vi "Calibration_user_input.vi"(4 "data mode":enum16{"Take new data point", "Refit Curve"}(ring), 6 "Mode":T5, 7 "Fixed n":bool, 8 "OK":T12, 9 "Sampling speeds":T6={"Samples /ch"=300, "Sampling Rate /ch (Hz)"=50.0} {"Sampling Rate /ch (Hz)" min=0 format="%.2f"; "Samples /ch" min=0 step=1}) -> (0 "Ch & Spans":T1[](array[typedef]) {"Ch No" min=0 max=7; "low limit (-10V)" min=-10 max=10 format="%.3f"; "high limit (10V)" min=-10 max=10 format="%.3f"}, 1 "Sampling speeds Output":T6={"Samples /ch"=300, "Sampling Rate /ch (Hz)"=50.0} {"Sampling Rate /ch (Hz)" min=0 format="%.2f"; "Samples /ch" min=0 step=1}, 2 "Fixed n out":bool, 3 "Temp (deg C)":dbl=21.0 format="%.1f", 5 "Abs Press (mbar)":dbl=1013.0 format="%.1f")   [LabVIEW 2013]
uses:
  Controls/ok_button.ctl
  Controls/TypeCalib.ctl
  Controls/Cal_Inst_type.ctl
  Controls/Calibration.ctl
  Calib_setup.ctl
  Controls/Ref_Inst_type.ctl
  Calib_mode.ctl
  Controls/PWA_Data.ctl
  File/Setup_Filetype.ctl
  Controls/Inst_type.ctl
  ADAM Client/Sub VIs/ADAM Controls/Channel_names.ctl
  Controls/LDA_Setup.ctl
  Controls/Setup.ctl
  Globals/Calib_global.vi
  Globals/Meas_global.vi
  Globals/LDA_meas_global_1.vi
  Globals/LDA_meas_global_2.vi
panel:
  in  "Acquisition Plug in":u16(ring) items=["ADAM_Server_Channels.vi", "Channels_and_Index.ctl", "DataTranslation.vi", "DT_With_Multiplexer.vi", "LDA_IP.vi", "NI-DAQmx.vi", "Simulate_kernal.vi"]
  in  "PWA Data":T2
  in  "Preston tube diammeter in mm":dbl min=0.0
  in  "Reference instrument Orig":T4={"high limit (10V)"=4.0, "low limit (-10V)"=0.0, "Ch No"=4, "Off ch no"=0, "Calib filename"=path "", "Ref Instrument type"=enum."Enter Value"} {"Off ch no" min=0 max=1; "Ch No" min=0 max=7; "low limit (-10V)" min=-10 max=10 format="%.1f"; "high limit (10V)" min=-10 max=10 format="%.1f"}
  out "Message":string
  in  "Ref Instrument type":T3
  out "Info":string
  out "XW Angle Calib Present?":bool
  out "XW Velocity Calib Present?":bool
  in  "Edit temp and Press":bool
  out "2nd ref instrument":T7={"2nd Ref type"=enum."LDA", "2nd inst present"=TRUE}
  in  "Ref vel for angle calib":T8={"high limit (10V)"=6.0, "low limit (-10V)"=0.0, "Ch No"=4, "Off ch no"=0, "Calib filename"=path "", "Ref Instrument type"=enum."LDA", "DAQmx Channel"=""} {"Off ch no" min=0 max=1; "Ch No" min=0 max=50; "low limit (-10V)" min=-10 max=10 format="%.1f"; "high limit (10V)" min=-10 max=10 format="%.1f"}
  out "Instrument type":T9=enum."Cross wire angle"
  in  "angle calib":T10(ring)
  in  "Reference instrument":T8={"high limit (10V)"=4.0, "low limit (-10V)"=0.0, "Ch No"=4, "Off ch no"=0, "Calib filename"=path "", "Ref Instrument type"=enum."Enter Value", "DAQmx Channel"=""} {"Off ch no" min=0 max=1; "Ch No" min=0 max=50; "low limit (-10V)" min=-10 max=10 format="%.1f"; "high limit (10V)" min=-10 max=10 format="%.1f"}
  in  "instrument to calibrate":T11=[{"high limit (10V)"=5.0, "low limit (-10V)"=3.0, "Ch No"=1, "Off ch no"=1, "DAQmx Channel"=""}, {"high limit (10V)"=5.0, "low limit (-10V)"=3.0, "Ch No"=2, "Off ch no"=1, "DAQmx Channel"=""}] {"Off ch no" min=0 max=1; "Ch No" min=0 max=1000; "low limit (-10V)" min=-10 max=10 format="%.3f"; "high limit (10V)" min=-10 max=10 format="%.3f"}
  in  "Instrument type":T9=enum."Pressure Transducer"
  out "Calib filename":path
  in  "Type":T1={"high limit (10V)"=4.0, "low limit (-10V)"=0.0, "Ch No"=4, "Var name"="LDA", "DAQmx Chan"=""} {"Ch No" min=0 max=7; "low limit (-10V)" min=-10 max=10 format="%.3f"; "high limit (10V)" min=-10 max=10 format="%.3f"}
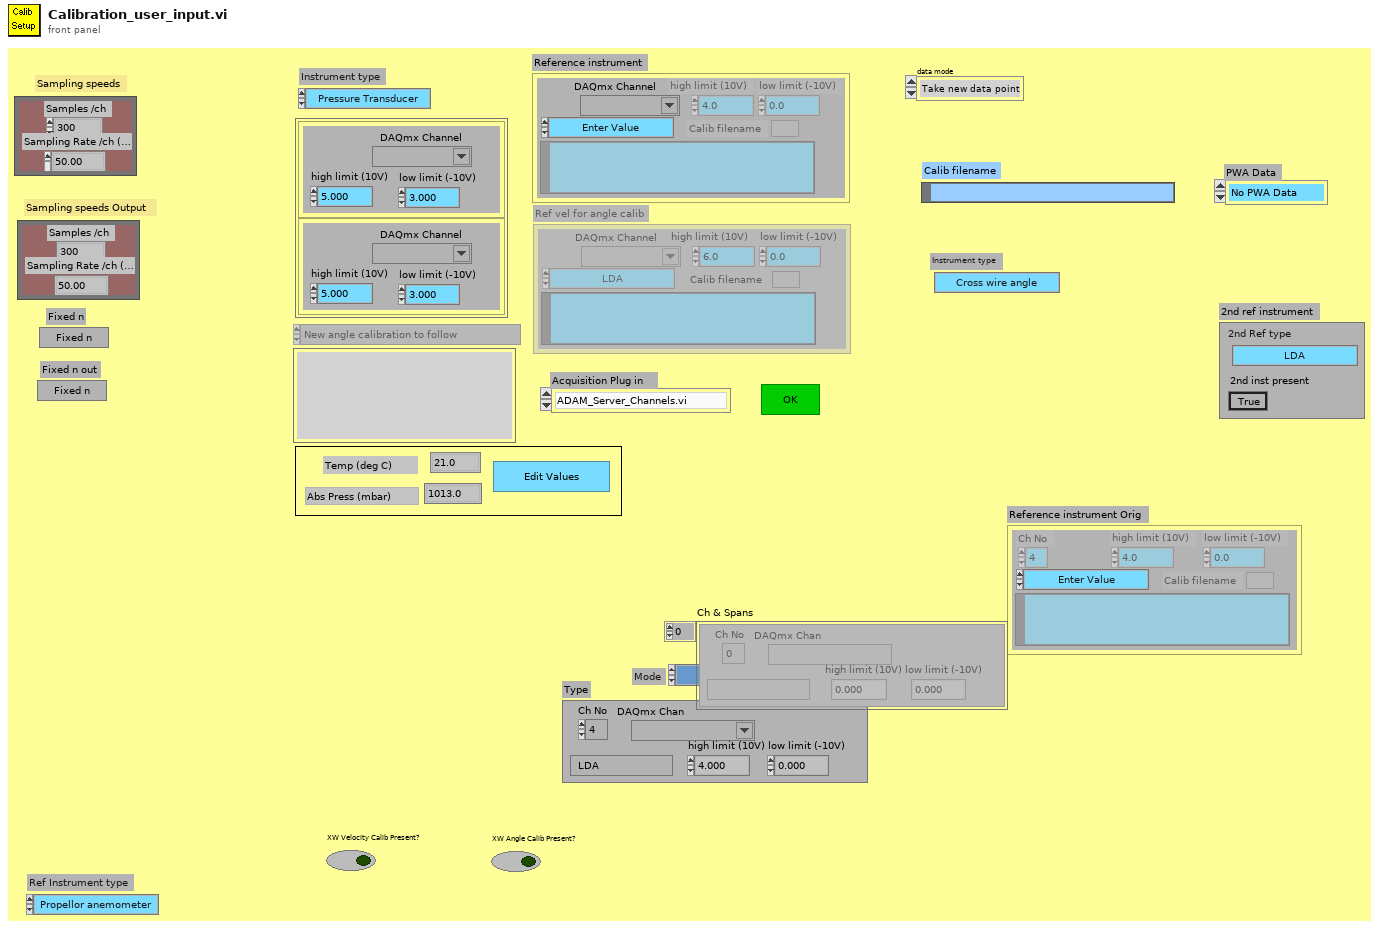
[diagram p1: front panel]
types:
  T1 = typedef "TypeCalib.ctl" = cluster{"high limit (10V)":sgl, "low limit (-10V)":sgl, "Ch No":i16, "Var name":string, "DAQmx Chan":tag}
  T2 = typedef "PWA_Data.ctl" = enum16{"No PWA Data", "One Ch PWA"}
  T3 = typedef "Ref_Inst_type.ctl" = enum16{"Propellor anemometer", "Pressure Transducer", "Raw voltage", "Pitot-static tube", "Preston tube", "Generic Linear", "Generic Polynomial", "Thermocouple", "LDA", "Enter Value", "ADAM Channel"}
  T4 = cluster{"high limit (10V)":sgl, "low limit (-10V)":sgl, "Ch No":i16, "Off ch no":i8, "Calib filename":path, "Ref Instrument type":T3}
  T5 = typedef "Calib_mode.ctl" = enum16{"Show Setup", "Take a New Calibration Point", "Refit Curve", "Setup Front Panel"}
  T6 = cluster{"Samples /ch":i32, "Sampling Rate /ch (Hz)":sgl}
  T7 = cluster{"2nd Ref type":T3, "2nd inst present":bool}
  T8 = typedef "Calib_setup.ctl" = cluster{"high limit (10V)":sgl, "low limit (-10V)":sgl, "Ch No":i16, "Off ch no":i8, "Calib filename":path, "Ref Instrument type":T3, "DAQmx Channel":tag}
  T9 = typedef "Cal_Inst_type.ctl" = enum16{"Propeller anemometer", "Pressure Transducer", "Hot wire", "Cross wire velocity", "Cross wire angle", "Generic Linear", "Generic Polynomial", "Generic BackPoly", "Fast FID", "Thermocouple", "Cold wire", "Pulsed Wire"}
  T10 = enum16{"New angle calibration to follow", "Use the most recent angle calibration"}
  T11 = typedef "Calibration.ctl" = cluster{"high limit (10V)":sgl, "low limit (-10V)":sgl, "Ch No":i16, "Off ch no":i8, "DAQmx Channel":tag}[]
  T12 = typedef "ok_button.ctl" = bool
  T13 = typedef "Setup_Filetype.ctl" = enum16{"Measurement Setups", "Calibration Setups", "General", "Results File Plotter Setups", "Speed Calib Tweaks"}
  T14 = typedef "Inst_type.ctl" = enum16{"Propeller anemometer", "Raw voltage", "Pressure Transducer", "Pitot-static tube", "Preston tube", "Hot wire", "Cross wire 1", "Cross wire 2", "Generic Linear", "Generic Polynomial", "Generic BackPoly", "Fast FID", "Thermocouple", "Cold wire", "Pulsed Wire", "LDA Vel", "LDA Tran time", "LDA Arr time"}
  T15 = typedef "Channel_names.ctl" = enum16{"Active Only", "Active + Off", "All Channels"}
  T16 = typedef "LDA_Setup.ctl" = cluster{"dimensions":enum16{"1D", "2D"}, "Analogue Freq Multiplier":dbl}
  T17 = typedef "Setup.ctl" = enum16{"Run Program", "Show Setup", "Save Current Setup", "Setup Front Panel"}
  T18 = cluster{"high limit (10V)":sgl, "low limit (-10V)":sgl, "Ch No":i16, "Off ch no":i8, "DAQmx Channel":tag}
  T19 = typedef "BSA_Type.ctl" = enum16{"57N11", "BSA F60"}
  T20 = typedef "BSA_info_Cluster.ctl" = cluster{"GPIB Address":string, "No of Check Bytes":i32, "Extra Info":string, "COLOUR":u32, "Wavelength (nm)":dbl}
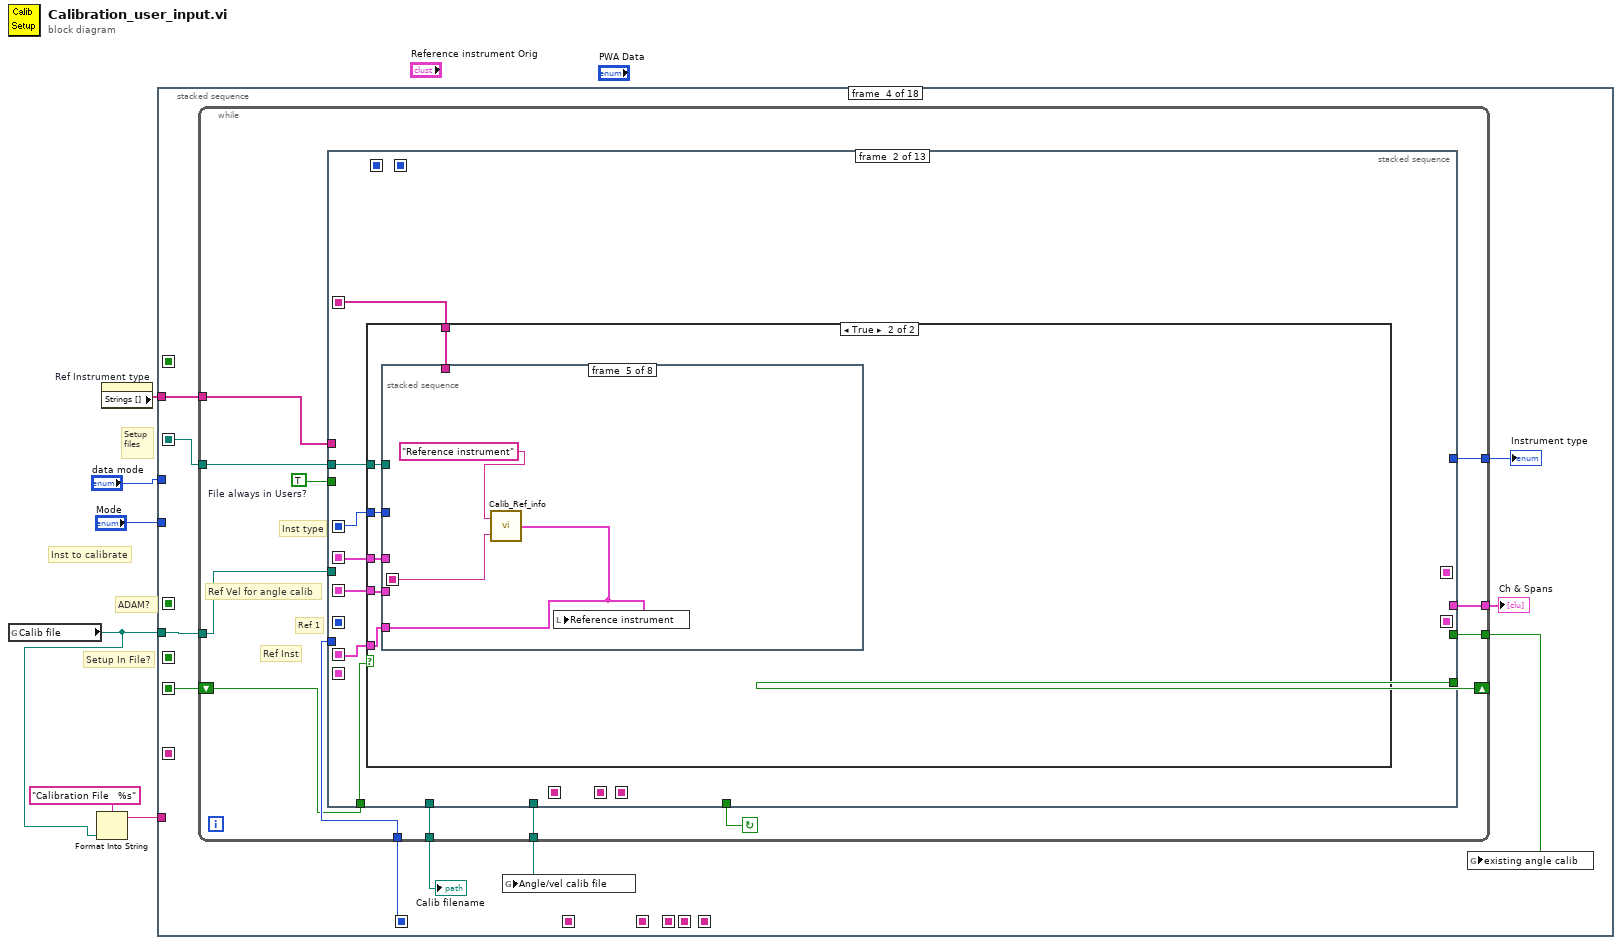
[diagram p0: block diagram]
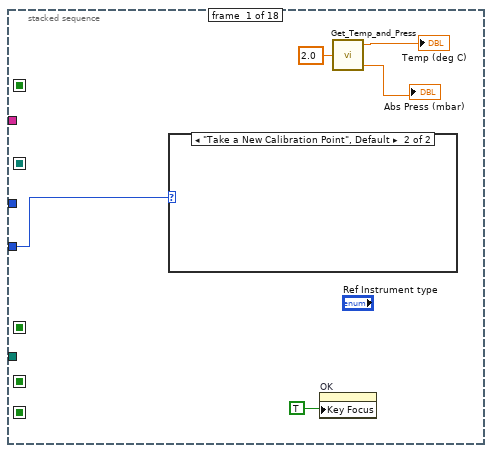
[diagram p2: hidden frame]
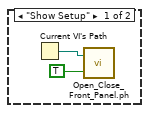
[diagram p3: hidden frame]
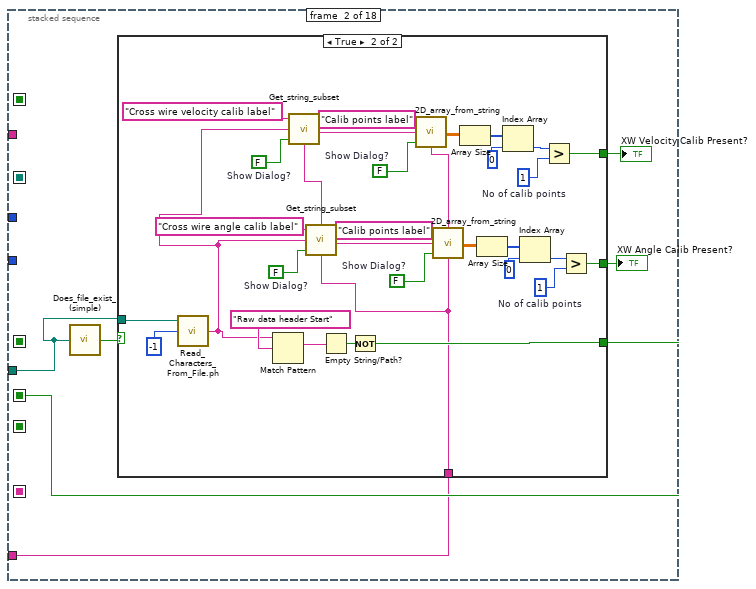
[diagram p4: hidden frame]
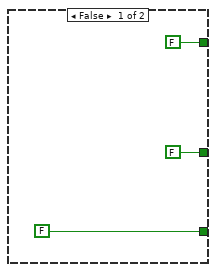
[diagram p5: hidden frame]
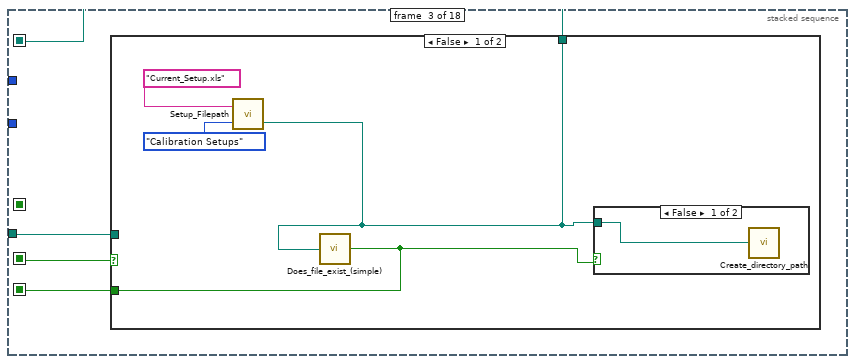
[diagram p6: hidden frame]
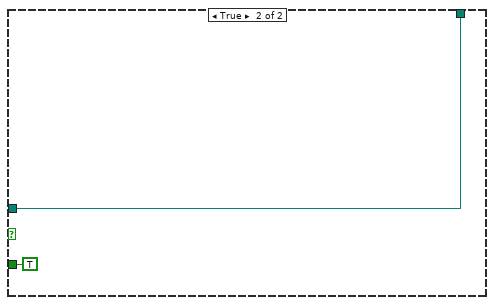
[diagram p8: hidden frame]
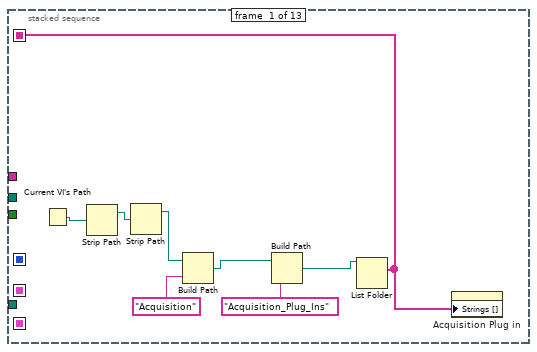
[diagram p9: hidden frame]
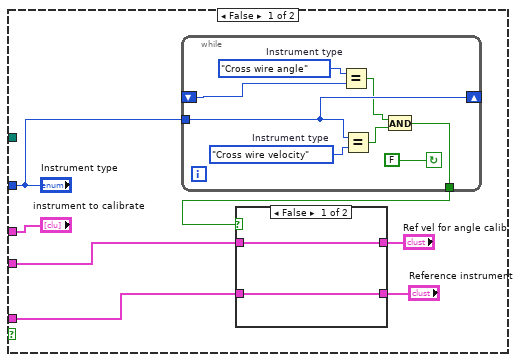
[diagram p10: hidden frame]
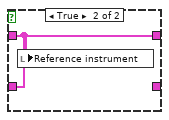
[diagram p11: hidden frame]
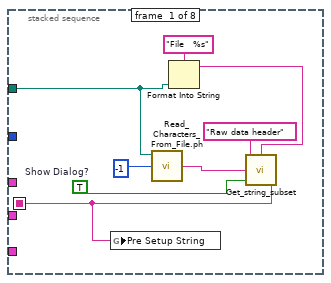
[diagram p12: hidden frame]
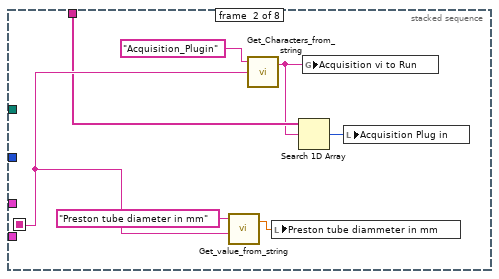
[diagram p13: hidden frame]
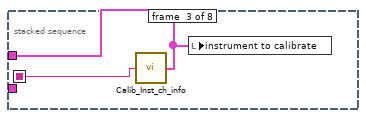
[diagram p14: hidden frame]
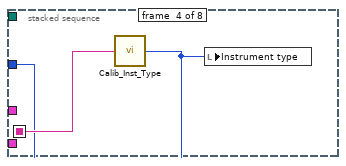
[diagram p15: hidden frame]
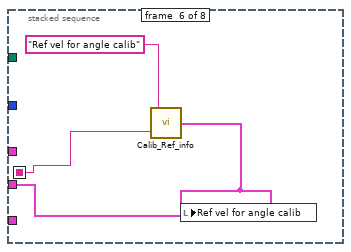
[diagram p16: hidden frame]
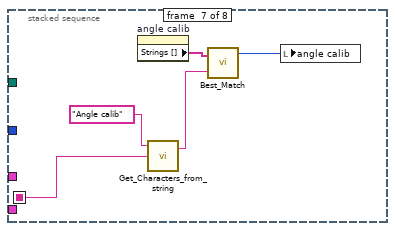
[diagram p17: hidden frame]
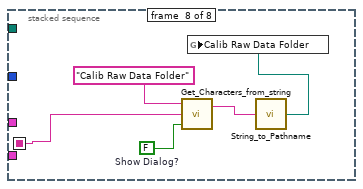
[diagram p18: hidden frame]
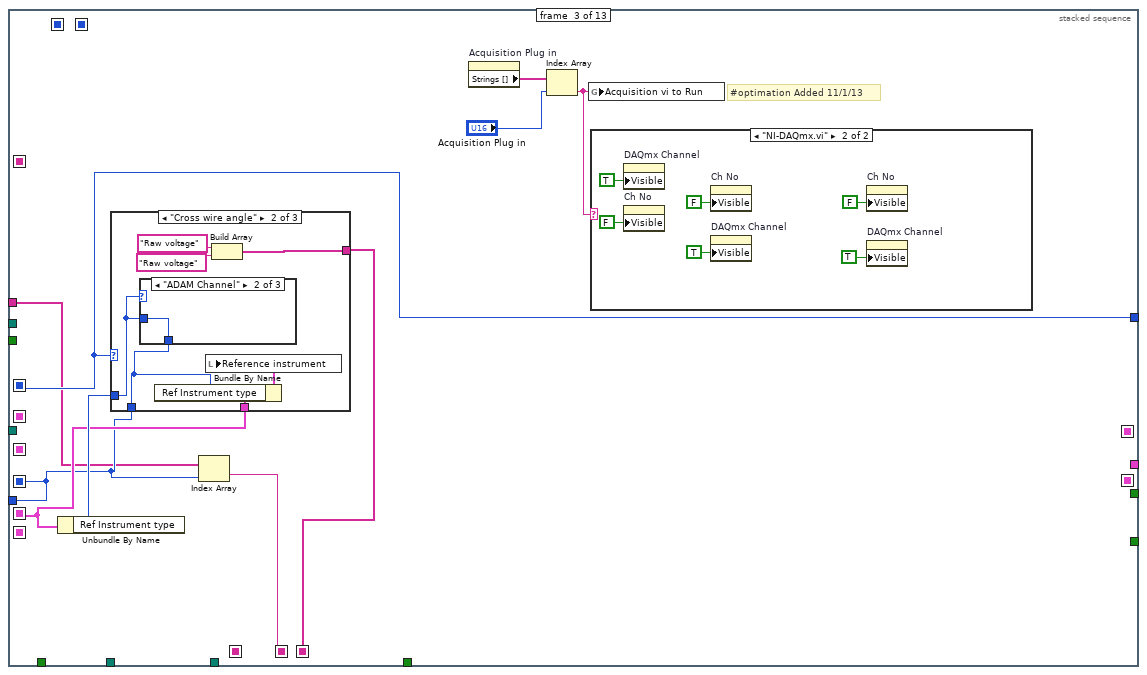
[diagram p19: hidden frame]
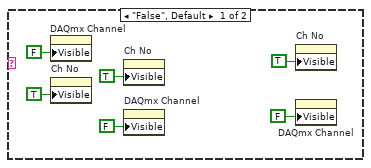
[diagram p20: hidden frame]
diagram:
  # "Inst to calibrate"
  # "Setup In File?"
  # "Setup\nfiles"
  # "ADAM?"
  n1 = global read "Calib_global.vi" "Calib file"() -> (w2:path)
  n2 = Format Into String(format string="Calibration File   %s", w2) -> (resulting string=w1:string)  [unwired: 2 in, 1 out]
  n3 = property on="Ref Instrument type" class="Enum (strict)"() -> ("Strings []"=w4:string[])  [unwired: 2 in, 2 out]
  n4 = stacked-sequence {
    seq-local: [_ _ w55 _ _ _ _ _ _ _ _ _ _ _ _ _ _ _] -> [_ _ _ w72 _ _ _ _ _ _ _ _ _ _ _ _ _ _]
    seq-local: [_ _ w56 _ _ _ _ _ _ _ _ _ _ _ _ _ _ _] -> [_ _ _ w70 _ _ _ _ _ _ _ _ _ _ _ _ _ _]
    seq-local: [_ _ _ w69 _ _ _ _ _ _ _ _ _ _ _ _ _ _] -> [_ _ _ _ _ _ _ w627 _ _ _ _ _ _ _ _ _ _]
    seq-local: [_ _ _ _ _ _ _ w628 _ _ _ _ _ _ _ _ _ _] -> [_ _ _ _ _ _ _ _ w645 _ _ _ _ _ _ _ _ _]
    seq-local: [_ _ _ _ _ _ _ _ w648 _ _ _ _ _ _ _ _ _] -> [_ _ _ _ _ _ _ _ _ _ _ _ _ _ w828 _ _ _]
    seq-local: [_ _ _ _ _ _ _ _ _ _ w737 _ _ _ _ _ _ _] -> [_ _ _ _ _ _ _ _ _ _ _ _ _ _ w827 _ w865 _]
    seq-local: [_ _ _ _ _ _ _ _ _ _ w734 _ _ _ _ _ _ _] -> [_ _ _ _ _ _ _ _ _ _ _ _ _ _ _ w834 _ _]
    seq-local: [_ w19 _ _ _ _ _ _ _ _ _ _ _ _ _ _ _ _] -> [_ _ w54 _ _ _ _ _ _ _ _ _ _ _ _ _ _ _]
    seq-local: [_ _ _ _ _ _ _ _ _ _ _ w749 _ _ _ _ _ _] -> [_ _ _ _ _ _ _ _ _ _ _ _ _ _ w820 _ _ _]
    seq-local: [_ _ _ _ _ _ _ _ _ _ _ _ _ w774 _ _ _ _] -> [_ _ _ _ _ _ _ _ _ _ _ _ _ _ w808 _ _ _]
    seq-local: [_ _ _ _ _ _ _ _ _ _ _ _ w756 _ _ _ _ _] -> [_ _ _ _ _ _ _ _ _ _ _ _ _ _ w804 _ w856 _]
    seq-local: [_ _ _ _ _ _ _ _ _ w683 _ _ _ _ _ _ _ _] -> [_ _ _ _ _ _ _ _ _ _ _ _ _ _ w803 _ _ _]
    tunnel: "Mode" -> [w7 _ _ _ w550 w568 _ _ w647 w696 _ _ w757 _ _ w836 _ w882]
    tunnel: "data mode" -> [_ _ _ _ w544 _ _ _ _ _ _ _ _ _ _ _ _ _]
    tunnel: w2 -> [_ w17 w53 w66 _ _ _ _ _ _ _ _ _ _ _ _ _ _]
    tunnel: w4 -> [_ _ _ w65 _ _ _ _ _ _ _ _ _ _ _ _ _ _]
    tunnel: w1 -> [_ w14 _ _ _ _ _ _ _ _ _ _ _ _ _ _ _ _]
    frame #0 {
      n5 = case shown="\"Take a New Calibration Point\", Default" w7 {
        frame "Show Setup" {
          n6 = Current VI's Path() -> (path=w13:path)
          n7 = call "Open_Close_Front_Panel.ph.vi"("Front Panel Window:Open"=TRUE, "VI path"=w13) -> ()  [unwired: 2 out]
        }
        frame "Take a New Calibration Point", Default {
        }
      }
      n8 = property on="OK" class="Bool"("Key Focus"=TRUE) -> ()  [unwired: 2 in, 2 out]
      n9 = call "Get_Temp_and_Press.vi"("Averaging time (mins)"=2.0) -> ("Abs Press (mbar)"=→"Abs Press (mbar)":dbl, "Temperature"=→"Temp (deg C)":dbl)  [unwired: 3 out]
    }
    frame #1 {
      n10 = call "Does_file_exist_(simple).vi"("Pathname"=w17) -> ("exists?"=w18:bool)
      n11 = case shown="True" w18 {
        tunnel: [FALSE w48] -> w19
        tunnel: w17 -> [_ w47]
        tunnel: [FALSE w25] -> w16
        tunnel: [FALSE w24] -> w15
        tunnel: w14 -> [_ w23]
        frame False {
        }
        frame True {
          w36 = 1  # No of calib points
          w30 = FALSE  # Show Dialog?
          w28 = FALSE  # Show Dialog?
          w37 = 1  # No of calib points
          w43 = FALSE  # Show Dialog?
          w45 = FALSE  # Show Dialog?
          n12 = call "Read_Characters_From_File.ph.vi"("file path (dialog if empty)"=w47, "number of characters (all:-1)"=-1) -> ("character string"=w26:string)  [unwired: 7 out]
          n13 = Match Pattern(string=w26, regular expression="Raw data header Start") -> (match substring=w50:string)  [unwired: 4 out]
          n14 = call "Get_string_subset.vi"("String Name"=w23, "Show Dialog?"=w28, "String to split"=w26, "File Label"="Cross wire velocity calib label") -> ("Output string"=w34:string)  [unwired: 1 out]
          n15 = call "Get_string_subset.vi"("String Name"=w23, "Show Dialog?"=w45, "String to split"=w26, "File Label"="Cross wire angle calib label") -> ("Output string"=w39:string)  [unwired: 1 out]
          n16 = Empty String/Path?(string/path=w50) -> (empty?=w49:bool)
          n17 = Not(x=w49) -> (.not. x?=w48:bool)
          n18 = call "2D_array_from_string.vi"("String Name"=w23, "Show Dialog?"=w30, "Input string"=w34, "Array title"="Calib points label") -> ("2D data array"=w31:dbl[][])
          n19 = call "2D_array_from_string.vi"("String Name"=w23, "Show Dialog?"=w43, "Input string"=w39, "Array title"="Calib points label") -> ("2D data array"=w42:dbl[][])
          n20 = Array Size(array=w31) -> (size(s)=w32:i32[])
          n21 = Array Size(array=w42) -> (size(s)=w41:i32[])
          n22 = Index Array(array=w32, index=0 ("Index")) -> (element=w35:i32)
          n23 = Index Array(array=w41, index=0 ("Index")) -> (element=w38:i32)
          n24 = Greater?(x=w35, y=w36) -> (0:w24:bool)
          n25 = Greater?(x=w38, y=w37) -> (0:w25:bool)
        }
      }
      "XW Velocity Calib Present?" <- w15
      "XW Angle Calib Present?" <- w16
    }
    frame #2 {
      n26 = case shown="False" w54 {
        tunnel: [w60 TRUE ("exists")] -> w56
        tunnel: [w57 w63] -> w55
        tunnel: w53 -> [_ w63]
        frame False {
          n27 = call "Setup_Filepath.vi"("Setup File Type"=Setup_Filetype."Calibration Setups", "Filename in"="Current_Setup.xls") -> ("Filename Out"=w57:path)  [unwired: 1 out]
          n28 = call "Does_file_exist_(simple).vi"("Pathname"=w57) -> ("exists?"=w60:bool)
          n29 = case shown="False" w60 {
            tunnel: w57 -> [w61 _]
            frame False {
              n30 = call "Create_directory_path.vi"("Path name"=w61) -> ()  [unwired: 1 in, 2 out]
            }
            frame True {
            }
          }
        }
        frame True {
        }
      }
    }
    frame #3 {
      n31 = while {
        tunnel: w65 -> [w77]
        shift-left: w70 -> [w80]
        shift-right: [w79] -> _
        tunnel: [w81] -> w71
        tunnel: w72 -> [w82]
        tunnel: [w83] -> w68
        tunnel: [w84] -> w64
        tunnel: [w85] -> w69
        tunnel: [w86] -> w73
        tunnel: [w75] -> w67
        tunnel: w66 -> [w74]
        stop <- w78 continue-if-true
        w76 = TRUE  # File always in Users?
        # "Ref 1"
        # "Ref Inst"
        # "Ref Vel for angle calib"
        # "Inst type"
        n32 = stacked-sequence {
          seq-local: [_ _ w166 _ _ _ _ _ _ _ _ _ _] -> [_ _ _ _ _ w294 _ _ _ _ _ _ _]
          seq-local: [_ _ w170 _ _ _ _ _ _ _ _ _ _] -> [_ _ _ _ _ _ _ _ w445 _ _ _ _]
          seq-local: [_ _ _ _ _ w288 _ _ _ _ _ _ _] -> [_ _ _ _ _ _ _ _ _ w463 _ _ _]
          seq-local: [_ _ w165 _ _ _ _ _ _ _ _ _ _] -> [_ _ _ _ _ _ _ _ _ w461 _ _ _]
          seq-local: [_ _ _ _ _ _ _ _ w444 _ _ _ _] -> [_ _ _ _ _ _ _ _ _ w462 _ _ _]
          seq-local: [_ _ _ _ _ _ _ w366 _ _ _ _ _] -> [_ _ _ _ _ _ _ _ _ w458 _ _ _]
          seq-local: [_ _ _ _ _ _ w362 _ _ _ _ _ _] -> [_ _ _ _ _ _ _ _ _ w457 _ _ _]
          seq-local: [_ w99 _ _ _ _ _ _ _ _ _ _ _] -> [_ _ w168 w205 w218 _ _ w367 _ _ _ _ _]
          seq-local: [_ w98 _ _ _ _ _ _ _ _ _ _ _] -> [_ _ _ w204 _ _ _ _ _ _ _ _ _]
          seq-local: [_ w97 _ _ _ _ _ _ _ _ _ _ _] -> [_ _ _ _ _ _ w364 w368 _ w456 _ _ _]
          seq-local: [_ w96 _ _ _ _ _ _ _ _ _ _ _] -> [_ _ w167 _ _ _ _ _ _ w455 _ _ w543]
          seq-local: [_ _ _ _ _ _ _ _ _ w454 _ _ _] -> [_ _ _ _ _ _ _ _ _ _ _ w502 _]
          seq-local: [_ _ _ w200 _ _ _ _ _ _ _ _ _] -> [_ _ _ _ _ _ _ _ w443 _ _ _ _]
          seq-local: [w87 _ _ _ _ _ _ _ _ _ _ _ _] -> [_ w95 _ _ _ _ _ _ _ _ _ _ _]
          tunnel: [_ _ _ _ _ _ _ _ _ w460 _ _ _] -> w86
          tunnel: [_ _ w166 _ _ _ _ _ _ _ _ _ _] -> w85
          tunnel: [_ _ _ _ _ _ _ _ _ w454 _ _ _] -> w84
          tunnel: [_ _ _ _ w223 _ _ _ _ _ _ _ _] -> w83
          tunnel: w82 -> [_ w101 _ _ _ _ _ _ _ _ _ _ _]
          tunnel: [_ _ w168 _ _ _ _ _ _ _ _ _ _] -> w81
          tunnel: w80 -> [_ w100 _ _ _ _ _ _ _ _ _ _ _]
          tunnel: [_ _ _ _ _ _ _ _ _ _ _ FALSE _] -> w79
          tunnel: [_ _ _ _ _ _ _ _ _ _ _ w500 _] -> w78
          tunnel: w77 -> [_ _ w164 _ _ _ w361 _ _ _ _ _ _]
          tunnel: w76 -> [_ _ _ _ _ _ _ _ _ _ _ _ _]
          tunnel: [_ _ _ _ w222 _ _ _ _ _ _ _ _] -> w75
          tunnel: w74 -> [_ _ _ _ w224 _ _ _ _ _ _ _ _]
          frame #0 {
            n33 = Current VI's Path() -> (path=w90:path)
            n34 = Strip Path(path=w90) -> (stripped path=w89:path)  [unwired: 1 out]
            n35 = Strip Path(path=w89) -> (stripped path=w88:path)  [unwired: 1 out]
            n36 = Build Path(base path=w88, name or relative path="Acquisition") -> (appended path=w93:path)
            n37 = Build Path(base path=w93, name or relative path="Acquisition_Plug_Ins") -> (appended path=w94:path)
            n38 = List Folder(path=w94) -> (filenames=w87:string[])  [unwired: 3 in, 3 out]
            n39 = property on="Acquisition Plug in" class="Ring (strict)"("Strings []"=w87) -> ()  [unwired: 2 in, 2 out]
          }
          frame #1 {
            n40 = case shown="True" w100 {
              tunnel: w101 -> [_ w125]
              tunnel: ["Instrument type" w123] -> w99
              tunnel: ["instrument to calibrate" w124] -> w98
              tunnel: [w103 w121] -> w97
              tunnel: [w105 w122] -> w96
              tunnel: w95 -> [_ w120]
              frame False {
                n41 = while {
                  shift-right: [w117] -> _
                  shift-left: _ -> [w115]
                  tunnel: "Instrument type" -> [w117]
                  tunnel: [w112] -> w106
                  stop <- FALSE continue-if-true
                  w116 = Cal_Inst_type."Cross wire angle"  # Instrument type
                  w118 = Cal_Inst_type."Cross wire velocity"  # Instrument type
                  n42 = Equal?(x=w116, y=w115) -> (x = y?=w113:bool)
                  n43 = Equal?(x=w117, y=w118) -> (x = y?=w114:bool)
                  n44 = And(x=w113, y=w114) -> (x .and. y?=w112:bool)
                }
                n45 = case shown="False" w106 {
                  tunnel: [w110 w111] -> w105
                  tunnel: "Reference instrument" -> [w110 _]
                  tunnel: [w109 w111] -> w103
                  tunnel: "Ref vel for angle calib" -> [w109 w111]
                  frame False {
                  }
                  frame True {
                    n46 = local write "Reference instrument"(w111) -> ()
                  }
                }
              }
              frame True {
                n47 = stacked-sequence {
                  seq-local: [w130 _ _ _ _ _ _ _] -> [_ w137 w142 w144 w146 w149 w153 w158]
                  tunnel: w125 -> [w127 _ _ _ _ _ _ _]
                  tunnel: [_ _ w141 _ _ _ _ _] -> w124
                  tunnel: [_ _ _ w143 _ _ _ _] -> w123
                  tunnel: [_ _ _ _ w145 _ _ _] -> w122
                  tunnel: [_ _ _ _ _ w148 _ _] -> w121
                  tunnel: w120 -> [_ w136 _ _ _ _ _ _]
                  frame #0 {
                    w129 = TRUE  # Show Dialog?
                    n48 = call "Read_Characters_From_File.ph.vi"("file path (dialog if empty)"=w127, "number of characters (all:-1)"=-1) -> ("character string"=w133:string)  [unwired: 7 out]
                    n49 = Format Into String(format string="File   %s", w127) -> (resulting string=w126:string)  [unwired: 2 in, 1 out]
                    n50 = call "Get_string_subset.vi"("String Name"=w126, "Show Dialog?"=w129, "String to split"=w133, "File Label"="Raw data header") -> ("Output string"=w130:string)  [unwired: 1 out]
                    n51 = global write "Calib_global.vi" "Pre Setup String"(w130) -> ()
                  }
                  frame #1 {
                    n52 = call "Get_value_from_string.vi"("Input string"=w137, "Variable name"="Preston tube diameter in mm") -> ("Value"=w139:dbl)  [unwired: 1 in, 1 out]
                    n53 = call "Get_Characters_from_string.vi"("Input string"=w137, "Variable name"="Acquisition_Plugin") -> ("Value"=w135:string)  [unwired: 1 in, 1 out]
                    n54 = local write "Preston tube diammeter in mm"(w139) -> ()
                    n55 = Search 1D Array(1D array=w136, element=w135) -> (index of element=w134:i32)  [unwired: 1 out]
                    n56 = global write "Meas_global.vi" "Acquisition vi to Run"(w135) -> ()
                    n57 = local write "Acquisition Plug in"(w134) -> ()
                  }
                  frame #2 {
                    n58 = call "Calib_Inst_ch_info.vi"("Input string"=w142) -> ("instrument to calibrate (new)"=w141:T11)
                    n59 = local write "instrument to calibrate"(w141) -> ()
                  }
                  frame #3 {
                    n60 = call "Calib_Inst_Type.vi"("Input string"=w144) -> ("Instrument type"=w143:T9)
                    n61 = local write "Instrument type"(w143) -> ()
                  }
                  frame #4 {
                    n62 = call "Calib_Ref_info.vi"("Input string"=w146, "Reference Name"="Reference instrument") -> ("Reference instrument"=w145:T8)
                    n63 = local write "Reference instrument"(w145) -> ()
                  }
                  frame #5 {
                    n64 = call "Calib_Ref_info.vi"("Input string"=w149, "Reference Name"="Ref vel for angle calib") -> ("Reference instrument"=w148:T8)
                    n65 = local write "Ref vel for angle calib"(w148) -> ()
                  }
                  frame #6 {
                    n66 = property on="angle calib" class="Enum (strict)"() -> ("Strings []"=w155:string[])  [unwired: 2 in, 2 out]
                    n67 = call "Get_Characters_from_string.vi"("Input string"=w153, "Variable name"="Angle calib") -> ("Value"=w152:string)  [unwired: 1 in, 1 out]
                    n68 = call "Best_Match.vi"("Input String"=w152, "String Options"=w155) -> ("index of element"=w151:i32)  [unwired: 1 out]
                    n69 = local write "angle calib"(w151) -> ()
                  }
                  frame #7 {
                    w159 = FALSE  # Show Dialog?
                    n70 = call "Get_Characters_from_string.vi"("Show Dialog?"=w159, "Input string"=w158, "Variable name"="Calib Raw Data Folder") -> ("Value"=w157:string)  [unwired: 1 out]
                    n71 = call "String_to_Pathname.vi"("Input String"=w157) -> ("path"=w156:path)
                    n72 = global write "Calib_global.vi" "Calib Raw Data Folder"(w156) -> ()
                  }
                }
              }
            }
          }
          frame #2 {
            # "#optimation Added 11/1/13"
            n73 = Unbundle By Name(w167) -> ("Ref Instrument type"=w169:T3)
            n74 = case shown="\"Cross wire angle\"" w168 {
              tunnel: [w185 w193 w198] -> w170
              tunnel: w169 -> [w183 w187 w197]
              tunnel: [w183 w190 w197] -> w166
              tunnel: w167 -> [_ w191 _]
              frame "Cross wire velocity" {
                n75 = Build Array("Raw voltage", "Raw voltage") -> (w185:string[])
              }
              frame "Cross wire angle" {
                n76 = case shown="\"ADAM Channel\"" w187 {
                  tunnel: [w194 w195 Ref_Inst_type."Enter Value" ("Ref Instrument type")] -> w190
                  tunnel: w187 -> [w194 w195 _]
                  frame "Enter Value" {
                  }
                  frame "ADAM Channel" {
                  }
                  frame "LDA", Default {
                  }
                }
                n77 = Bundle By Name(cluster=w191, "Ref Instrument type"=w190) -> (w192:T8)
                n78 = local write "Reference instrument"(w192) -> ()
                n79 = Build Array("Raw voltage", "Raw voltage") -> (w193:string[])
              }
              frame "Generic Linear", Default {
                n80 = Build Array("Raw voltage") -> (w198:string[])
              }
            }
            n81 = Index Array(array=w164, index=w166) -> (element=w165:string)
            n82 = property on="Acquisition Plug in" class="Ring (strict)"() -> ("Strings []"=w163:string[])  [unwired: 2 in, 2 out]
            n83 = Index Array(array=w163, index="Acquisition Plug in") -> (element=w161:string)
            n84 = global write "Meas_global.vi" "Acquisition vi to Run"(w161) -> ()
            n85 = case shown="\"NI-DAQmx.vi\"" w161 {
              frame "False", Default {
                n86 = property on="DAQmx Channel" class="DAQmxName"("Visible"=FALSE) -> ()  [unwired: 2 in, 2 out]
                n87 = property on="Ch No" class="DigNum (strict)"("Visible"=TRUE) -> ()  [unwired: 2 in, 2 out]
                n88 = property on="Ch No" class="DigNum (strict)"("Visible"=TRUE) -> ()  [unwired: 2 in, 2 out]
                n89 = property on="DAQmx Channel" class="DAQmxName"("Visible"=FALSE) -> ()  [unwired: 2 in, 2 out]
                n90 = property on="Ch No" class="DigNum (strict)"("Visible"=TRUE) -> ()  [unwired: 2 in, 2 out]
                n91 = property on="DAQmx Channel" class="DAQmxName"("Visible"=FALSE) -> ()  [unwired: 2 in, 2 out]
              }
              frame "NI-DAQmx.vi" {
                n92 = property on="DAQmx Channel" class="DAQmxName"("Visible"=TRUE) -> ()  [unwired: 2 in, 2 out]
                n93 = property on="Ch No" class="DigNum (strict)"("Visible"=FALSE) -> ()  [unwired: 2 in, 2 out]
                n94 = property on="Ch No" class="DigNum (strict)"("Visible"=FALSE) -> ()  [unwired: 2 in, 2 out]
                n95 = property on="DAQmx Channel" class="DAQmxName"("Visible"=TRUE) -> ()  [unwired: 2 in, 2 out]
                n96 = property on="Ch No" class="DigNum (strict)"("Visible"=FALSE) -> ()  [unwired: 2 in, 2 out]
                n97 = property on="DAQmx Channel" class="DAQmxName"("Visible"=TRUE) -> ()  [unwired: 2 in, 2 out]
              }
            }
          }
          frame #3 {
            n98 = Array Size(array=w204) -> (size(s)=w203:i32)
            n99 = case shown="\"Cross wire angle\"" w205 {
              tunnel: [2 2 1 0] -> w202
              frame "Cross wire velocity" {
              }
              frame "Cross wire angle" {
              }
              frame "Generic Linear", Default {
              }
              frame "Pulsed Wire" {
              }
            }
            n100 = Equal?(x=w202, y=w203) -> (x = y?=w201:bool)
            n101 = case shown="False" w201 {
              tunnel: w202 -> [w211 _]
              tunnel: w204 -> [w207 w213]
              tunnel: [w206 w213] -> w200
              frame False {
                n102 = Index Array(array=w207, index=0) -> (element=w208:T18)
                n103 = Build Array (concatenate)(w207, w208) -> (w210:T11)
                n104 = for {
                  N: w211 -> [_]
                  tunnel: w210 -> [w212] mode=indexing
                  tunnel: [w212] -> w206 mode=indexing
                }
                n105 = local write "instrument to calibrate"(w206) -> ()
              }
              frame True {
              }
            }
          }
          frame #4 {
            n106 = case shown="\"Cross wire angle\"" w218 {
              tunnel: w224 -> [_ w235 w257]
              tunnel: [path "" w236 w258] -> w223
              tunnel: [FALSE w234 w256] -> w222
              tunnel: [w225 w230 w252] -> w221
              tunnel: [w227 w233 w255] -> w220
              tunnel: ["" w232 w253] -> w219
              tunnel: w218 -> [_ w231 w254]
              frame "Propeller anemometer", Default {
                w225 = u8 2  # Disabled
                w227 = u8 2  # Disabled
              }
              frame "Cross wire angle" {
                w230 = u8 0  # Disabled
                w233 = u8 2  # Disabled
                n107 = local read "XW Velocity Calib Present?"() -> (w237:bool)
                n108 = case shown="False" w237 {
                  tunnel: [w241 w251] -> w236
                  tunnel: w235 -> [_ w251]
                  tunnel: [TRUE TRUE] -> w234
                  tunnel: [w239 w249] -> w232
                  tunnel: w231 -> [w238 _]
                  frame False {
                    w245 = 0  # index
                    n109 = local read "instrument to calibrate"() -> (w246:T11)
                    n110 = Index Array(array=w246, index=w245) -> (element=w244:T18)
                    n111 = Unbundle By Name(w244) -> ("Ch No"=w242:i16)
                    n112 = call "XW_file_info.vi"("Instrument type"=w238, "Ch No"=w242) -> ("Filename"=w241:path, "resulting string"=w239:string, "File Exists?"=w240:bool)
                    n113 = case shown="False" w240 {
                      frame False {
                        w247 = Cal_Inst_type."Cross wire velocity"  # Instrument type
                        w248 = "You need to do a velocity calibration before you can do the angle calibration"  # message
                        n114 = local write "Instrument type"(w247) -> ()
                        n115 = One Button Dialog(message=w248) -> ()  [unwired: 2 out]
                      }
                      frame True {
                      }
                    }
                  }
                  frame True {
                    w249 = "Will use the velocity Calibration info already in the Calibration file. "  # resulting string
                  }
                }
              }
              frame "Cross wire velocity" {
                w252 = u8 2  # Disabled
                n116 = local read "XW Angle Calib Present?"() -> (w259:bool)
                n117 = case shown="False" w259 {
                  tunnel: [w268 w287] -> w258
                  tunnel: w257 -> [_ w287]
                  tunnel: [TRUE FALSE] -> _
                  tunnel: [w267 TRUE] -> w256
                  tunnel: [w266 w284] -> w255
                  tunnel: w254 -> [w264 _]
                  tunnel: [w261 w283] -> w253
                  frame False {
                    w272 = 0  # index
                    n118 = local read "instrument to calibrate"() -> (w273:T11)
                    n119 = Index Array(array=w273, index=w272) -> (element=w271:T18)
                    n120 = Unbundle By Name(w271) -> ("Ch No"=w265:i16)
                    n121 = call "XW_file_info.vi"("Instrument type"=w264, "Ch No"=w265) -> ("Filename"=w263:path, "resulting string"=w260:string, "File Exists?"=w262:bool)
                    n122 = case shown="\"New angle calibration to follow\"" "angle calib" {
                      tunnel: [path "" w279] -> w268
                      tunnel: w263 -> [_ w279]
                      tunnel: [FALSE TRUE] -> w267
                      tunnel: ["This XW velocity Calibration MUST be followed by an angle calibration, before XW measurements can be made." w277] -> w261
                      tunnel: w260 -> [_ w277]
                      frame "New angle calibration to follow" {
                      }
                      frame "Use the most recent angle calibration" {
                      }
                    }
                    n123 = case shown="False" w262 {
                      tunnel: [w280 w282] -> w266
                      frame False {
                        w280 = u8 2  # Disabled
                        w281 = T10."New angle calibration to follow"  # angle calib
                        n124 = local write "angle calib"(w281) -> ()
                      }
                      frame True {
                        w282 = u8 0  # Disabled
                      }
                    }
                  }
                  frame True {
                    w283 = "Will use the angle Calibration info already in the Calibration file. "  # resulting string
                    w284 = u8 0  # Disabled
                  }
                }
              }
            }
            "Info" <- w219
            n125 = property on="Ref vel for angle calib" class="Clust (strict)"("Disabled"=w221) -> ()  [unwired: 2 in, 2 out]
            n126 = property on="angle calib" class="Enum (strict)"("Disabled"=w220) -> ()  [unwired: 2 in, 2 out]
          }
          frame #5 {
            n127 = case shown="\"Enter Value\"" w294 {
              tunnel: [u8 0 u8 0 u8 0 u8 0 u8 0 u8 0 u8 0 u8 2 u8 2 u8 2 u8 2] -> w289
              tunnel: [u8 0 u8 0 u8 2 u8 0 u8 0 u8 0 u8 0 u8 2 u8 2 u8 2 u8 2] -> w293
              tunnel: [u8 0 u8 0 u8 0 u8 0 u8 0 u8 0 u8 0 u8 2 u8 2 u8 2 u8 2] -> w292
              tunnel: [u8 0 u8 0 u8 0 u8 0 u8 0 u8 0 u8 0 u8 2 u8 2 u8 2 u8 2] -> w291
              tunnel: [u8 0 u8 0 u8 0 u8 0 u8 0 u8 0 u8 0 u8 2 u8 2 u8 2 u8 2] -> w290
              tunnel: [1 1 1 1 1 1 1 0 0 0 0] -> w288
              frame "Propellor anemometer" {
              }
              frame "Pressure Transducer" {
              }
              frame "Raw voltage" {
              }
              frame "Pitot-static tube" {
              }
              frame "Preston tube" {
              }
              frame "Generic Linear" {
              }
              frame "Generic Polynomial" {
              }
              frame "Thermocouple" {
              }
              frame "LDA" {
              }
              frame "Enter Value" {
              }
              frame "ADAM Channel" {
              }
            }
            n128 = property on="Calib filename" class="Path"("Disabled"=w293) -> ()  [unwired: 2 in, 2 out]
            n129 = property on="Ch No" class="DigNum (strict)"("Disabled"=w292) -> ()  [unwired: 2 in, 2 out]
            n130 = property on="high limit (10V)" class="DigNum (strict)"("Disabled"=w291) -> ()  [unwired: 2 in, 2 out]
            n131 = property on="low limit (-10V)" class="DigNum (strict)"("Disabled"=w290) -> ()  [unwired: 2 in, 2 out]
            n132 = property on="Off ch no" class="DigNum (strict)"("Disabled"=w289) -> ()  [unwired: 2 in, 2 out]
          }
          frame #6 {
            n133 = Unbundle By Name(w364) -> ("Ref Instrument type"=w363:T3)
            n134 = Index Array(array=w361, index=w363) -> (element=w362:string)
          }
          frame #7 {
            n135 = Unbundle By Name(w368) -> ("Ref Instrument type"=w369:T3)
            n136 = case shown="\"Pitot-static tube\"" w369 {
              tunnel: [u8 0 u8 0 u8 0 u8 0 u8 0 u8 0 u8 0 u8 0 u8 2 u8 2 u8 2] -> w370
              tunnel: [u8 0 u8 0 u8 2 u8 0 u8 0 u8 0 u8 0 u8 0 u8 2 u8 2 u8 2] -> w374
              tunnel: [u8 0 u8 0 u8 0 u8 0 u8 0 u8 0 u8 0 u8 0 u8 2 u8 2 u8 2] -> w373
              tunnel: [u8 0 u8 0 u8 0 u8 0 u8 0 u8 0 u8 0 u8 0 u8 2 u8 2 u8 2] -> w372
              tunnel: [u8 0 u8 0 u8 0 u8 0 u8 0 u8 0 u8 0 u8 0 u8 2 u8 2 u8 2] -> w371
              tunnel: [enum16{"No 2nd ref inst", "Add 2nd ref inst"}."Add 2nd ref inst" enum16{"No 2nd ref inst", "Add 2nd ref inst"}."Add 2nd ref inst" enum16{"No 2nd ref inst", "Add 2nd ref inst"}."Add 2nd ref inst" enum16{"No 2nd ref inst", "Add 2nd ref inst"}."Add 2nd ref inst" enum16{"No 2nd ref inst", "Add 2nd ref inst"}."Add 2nd ref inst" enum16{"No 2nd ref inst", "Add 2nd ref inst"}."Add 2nd ref inst" enum16{"No 2nd ref inst", "Add 2nd ref inst"}."Add 2nd ref inst" enum16{"No 2nd ref inst", "Add 2nd ref inst"}."Add 2nd ref inst" enum16{"No 2nd ref inst", "Add 2nd ref inst"}."No 2nd ref inst" enum16{"No 2nd ref inst", "Add 2nd ref inst"}."No 2nd ref inst" enum16{"No 2nd ref inst", "Add 2nd ref inst"}."No 2nd ref inst"] -> w365
              frame "Propellor anemometer" {
              }
              frame "Pressure Transducer" {
              }
              frame "Raw voltage" {
              }
              frame "Pitot-static tube" {
              }
              frame "Preston tube" {
              }
              frame "Generic Linear" {
              }
              frame "Generic Polynomial" {
              }
              frame "Thermocouple" {
              }
              frame "LDA" {
              }
              frame "Enter Value" {
              }
              frame "ADAM Channel" {
              }
            }
            n137 = case shown="\"Cross wire angle\"" w367 {
              tunnel: [w375 enum16{"No 2nd ref inst", "Add 2nd ref inst"}."No 2nd ref inst"] -> w366
              tunnel: w365 -> [w375 _]
              frame "Cross wire angle" {
              }
              frame "Generic Linear", Default {
              }
            }
            n138 = property on="Calib filename" class="Path"("Disabled"=w374) -> ()  [unwired: 2 in, 2 out]
            n139 = property on="low limit (-10V)" class="DigNum (strict)"("Disabled"=w373) -> ()  [unwired: 2 in, 2 out]
            n140 = property on="high limit (10V)" class="DigNum (strict)"("Disabled"=w372) -> ()  [unwired: 2 in, 2 out]
            n141 = property on="Ch No" class="DigNum (strict)"("Disabled"=w371) -> ()  [unwired: 2 in, 2 out]
            n142 = property on="Off ch no" class="DigNum (strict)"("Disabled"=w370) -> ()  [unwired: 2 in, 2 out]
          }
          frame #8 {
            n143 = for {
              tunnel: w445 -> [w453] mode=indexing
              tunnel: [w451] -> w444 mode=indexing
              tunnel: w443 -> [w447] mode=indexing
              n144 = Unbundle By Name(w447) -> ("high limit (10V)"=w450:sgl, "low limit (-10V)"=w449:sgl, "Ch No"=w448:i16, "DAQmx Channel"=w446:tag)
              n145 = Bundle By Name(cluster="Type", "high limit (10V)"=w450, "low limit (-10V)"=w449, "Ch No"=w448, "Var name"=w453, "DAQmx Chan"=w446) -> (w451:T1)
            }
          }
          frame #9 {
            n146 = local read "Type"() -> (w459:T1)
            n147 = case shown="..0" w463 {
              tunnel: [w467 w491] -> w454
              tunnel: w462 -> [w470 w485]
              tunnel: w455 -> [_ w488]
              tunnel: w461 -> [_ w487]
              tunnel: [w469 w490] -> w460
              tunnel: w459 -> [w468 w489]
              tunnel: w456 -> [w464 _]
              tunnel: w458 -> [w466 _]
              tunnel: w457 -> [w465 _]
              frame ..0 {
                n148 = case shown="\"Add 2nd ref inst\"" w466 {
                  tunnel: [w472 w483] -> w467
                  tunnel: w465 -> [_ w482]
                  tunnel: w464 -> [_ w481]
                  tunnel: w468 -> [_ w480]
                  tunnel: [path "" w479] -> w469
                  tunnel: w470 -> [w472 w474]
                  frame "No 2nd ref inst" {
                  }
                  frame "Add 2nd ref inst" {
                    n149 = Unbundle By Name(w481) -> ("high limit (10V)"=w476:sgl, "low limit (-10V)"=w477:sgl, "Ch No"=w478:i16, "Calib filename"=w479:path, "DAQmx Channel"=w473:tag)
                    n150 = Bundle By Name(cluster=w480, "high limit (10V)"=w476, "low limit (-10V)"=w477, "Ch No"=w478, "Var name"=w482, "DAQmx Chan"=w473) -> (w475:T1)
                    n151 = Build Array (concatenate)(w475, w474) -> (w483:T1[])
                  }
                }
              }
              frame 1.. {
                n152 = Unbundle By Name(w488) -> ("high limit (10V)"=w494:sgl, "low limit (-10V)"=w493:sgl, "Ch No"=w492:i16, "Calib filename"=w490:path, "DAQmx Channel"=w484:tag)
                n153 = Bundle By Name(cluster=w489, "high limit (10V)"=w494, "low limit (-10V)"=w493, "Ch No"=w492, "Var name"=w487, "DAQmx Chan"=w484) -> (w486:T1)
                n154 = local write "Type"(w486) -> ()
                n155 = Build Array (concatenate)(w486, w485) -> (w491:T1[])
              }
            }
          }
          frame #10 {
            n156 = case shown="True" "Edit temp and Press" {
              frame False {
              }
              frame True {
                n157 = stacked-sequence {
                  frame #0 {
                    w496 = TRUE  # Wait until done
                    n158 = call "Run_Enter_Temp.vi"("Wait until done"=w496) -> ()  [unwired: 1 out]
                  }
                  frame #1 {
                    n159 = call "Get_Temp_and_Press.vi"("Averaging time (mins)"=0.5) -> ("Abs Press (mbar)"=w498:dbl, "Temperature"=w497:dbl)  [unwired: 3 out]
                    n160 = local write "Abs Press (mbar)"(w498) -> ()
                    n161 = local write "Temp (deg C)"(w497) -> ()
                  }
                }
              }
            }
          }
          frame #11 {
            # "#optimation Should probably also check for duplicate DAQmx Channels"
            n162 = case shown="True" "OK" {
              tunnel: w502 -> [_ w506]
              tunnel: [TRUE w505] -> w500
              frame False {
              }
              frame True {
                n163 = stacked-sequence {
                  seq-local: [w507 _] -> [_ w525]
                  tunnel: w506 -> [w509 w527]
                  tunnel: [_ w523] -> w505
                  frame #0 {
                    n164 = for {
                      shift-right: [w516] -> _
                      shift-left: i16[] [] -> [w515]
                      tunnel: w509 -> [w512] mode=indexing
                      tunnel: [w511] -> w508 mode=indexing
                      n165 = Unbundle By Name(w512) -> ("Ch No"=w513:i16)
                      n166 = Search 1D Array(1D array=w515, element=w513) -> (index of element=w514:i32)  [unwired: 1 out]
                      n167 = Build Array (concatenate)(w515, w513) -> (w516:i16[])
                      n168 = case shown="0, Default" w514 {
                        tunnel: w513 -> [w521 _]
                        tunnel: [w517 FALSE ("true")] -> w511
                        frame 0, Default {
                          n169 = Format Into String(format string="The Ch No %d appears more than once", w521) -> (resulting string=w519:string)  [unwired: 2 in, 1 out]
                          n170 = One Button Dialog(message=w519, button name ("OK")="Ok") -> (true=w517:bool)
                        }
                        frame -1 {
                        }
                      }
                    }
                    n171 = Or Array Elements(Boolean array=w508) -> (logical OR=w507:bool)
                  }
                  frame #1 {
                    n172 = for {
                      tunnel: w527 -> [w533] mode=indexing
                      tunnel: [w532] -> w526 mode=indexing
                      n173 = Unbundle By Name(w533) -> ("high limit (10V)"=w531:sgl, "low limit (-10V)"=w530:sgl, "Ch No"=w528:i16)
                      n174 = Greater Or Equal?(x=w531, y=w530) -> (x >= y?=w529:bool)
                      n175 = case shown="False" w529 {
                        tunnel: [TRUE ("true") FALSE ("true")] -> w532
                        tunnel: w528 -> [w535 _]
                        frame False {
                          n176 = Number To Decimal String(number=w535) -> (decimal integer string=w536:string)  [unwired: 1 out]
                          n177 = Concatenate Strings("Error in input limits for Channel No ", w536) -> (w537:string)
                          n178 = One Button Dialog(message=w537) -> ()  [unwired: 2 out]
                        }
                        frame True {
                        }
                      }
                    }
                    n179 = Or Array Elements(Boolean array=w526) -> (logical OR=w524:bool)
                    n180 = Or(x=w524, y=w525) -> (x .or. y?=w523:bool)
                  }
                }
              }
            }
          }
          frame #12 {
            n181 = Unbundle By Name(w543) -> ("Ref Instrument type"=w542:T3)
            n182 = Equal?(x=Ref_Inst_type."Preston tube" ("Ref Instrument type"), y=w542) -> (x = y?=w540:bool)
            n183 = property on="Preston tube diammeter in mm" class="DigNum (strict)"("Visible"=w540) -> ()  [unwired: 2 in, 2 out]
          }
        }
      }
      "Instrument type" <- w71
      "Calib filename" <- w73
      "Ch & Spans" <- w64
      n184 = global write "Calib_global.vi" "Angle/vel calib file"(w68) -> ()
      n185 = global write "Calib_global.vi" "existing angle calib"(w67) -> ()
    }
    frame #4 {
      n186 = global read "Calib_global.vi" "Pre Setup String"() -> (w545:string)
      n187 = case shown="\"Setup Front Panel\"" w550 {
        tunnel: [w552 w562] -> w549
        tunnel: "Sampling speeds" -> [w552 w564]
        tunnel: [w551 w558] -> w547
        tunnel: "Fixed n" -> [w551 _]
        tunnel: w545 -> [_ w557]
        tunnel: w544 -> [_ _]
        frame "Show Setup", Default {
        }
        frame "Setup Front Panel" {
          n188 = call "Get_value_from_string.vi"("Input string"=w557, "Variable name"="Requested sampling rate") -> ("Status"=w555:enum16{"Char in string", "Char not in string"}, "Value"=w553:dbl)  [unwired: 1 in]
          n189 = case shown="\"Char not in string\"" w555 {
            tunnel: [w566 sgl 100.0 ("Sampling Rate /ch (Hz)")] -> w554
            tunnel: w553 -> [w566 _]
            frame "Char in string" {
            }
            frame "Char not in string" {
            }
          }
          n190 = call "Get_value_from_string.vi"("Input string"=w557, "Variable name"="No of samples") -> ("Value"=w563:dbl)  [unwired: 1 in, 1 out]
          n191 = call "Get_Characters_from_string.vi"("Input string"=w557, "Variable name"="Fixed Coefficient n") -> ("Value"=w560:string)  [unwired: 1 in, 1 out]
          n192 = Bundle By Name(cluster=w564, "Samples /ch"=w563, "Sampling Rate /ch (Hz)"=w554) -> (w562:T6)
          n193 = Equal?(x="TRUE", y=w560) -> (x = y?=w558:bool)
        }
      }
      "Sampling speeds Output" <- w549
      "Fixed n out" <- w547
    }
    frame #5 {
      n194 = property on="Calib filename" class="Path"() -> ("Disabled"=w572:u8)  [unwired: 2 in, 2 out]
      n195 = Equal To 0?(x=w572) -> (x = 0?=w571:bool)
      n196 = local read "Reference instrument"() -> (w570:T8)
      n197 = case shown="True" w571 {
        tunnel: w570 -> [w575 w581]
        tunnel: [w574 w580] -> w569
        tunnel: w568 -> [_ w576]
        frame False {
          n198 = Bundle By Name(cluster=w575, "Calib filename"=path "") -> (w574:T8)
        }
        frame True {
          w577 = FALSE  # Use Latest Calib
          n199 = Unbundle By Name(w581) -> ("Calib filename"=w583:path, "Ref Instrument type"=w579:T3)
          n200 = case shown="\"Generic Polynomial\"" w579 {
            tunnel: [Inst_type."Propeller anemometer" ("Inst type") Inst_type."Pressure Transducer" ("Inst type") Inst_type."Pressure Transducer" ("Inst type") Inst_type."Pitot-static tube" ("Inst type") Inst_type."Preston tube" ("Inst type") Inst_type."Generic Linear" ("Inst type") Inst_type."Generic Polynomial" ("Inst type") Inst_type."Thermocouple" ("Inst type") Inst_type."Raw voltage" ("Inst type") Inst_type."Raw voltage" ("Inst type") Inst_type."Raw voltage" ("Inst type")] -> w578
            frame "Propellor anemometer" {
            }
            frame "Pressure Transducer" {
            }
            frame "Raw voltage" {
            }
            frame "Pitot-static tube" {
            }
            frame "Preston tube" {
            }
            frame "Generic Linear" {
            }
            frame "Generic Polynomial" {
            }
            frame "Thermocouple" {
            }
            frame "LDA" {
            }
            frame "Enter Value" {
            }
            frame "ADAM Channel" {
            }
          }
          n201 = case shown="\"Take a New Calibration Point\", Default" w576 {
            tunnel: w583 -> [w584 w588]
            tunnel: [w584 w587] -> w582
            tunnel: w578 -> [_ w586]
            tunnel: w577 -> [_ w585]
            frame "Refit Curve" {
            }
            frame "Take a New Calibration Point", Default {
              n202 = call "Find_calibration_file.vi"("Inst type"=w586, "Use Latest Calib"=w585, "filename"=w588) -> ("filename out"=w587:path)  [unwired: 1 in]
            }
          }
          n203 = Bundle By Name(cluster=w581, "Calib filename"=w582) -> (w580:T8)
        }
      }
      n204 = local write "Reference instrument"(w569) -> ()
    }
    frame #6 {
      n205 = property on="Ref vel for angle calib" class="Clust (strict)"() -> ("Disabled"=w600:u8)  [unwired: 2 in, 2 out]
      n206 = local read "Ref vel for angle calib"() -> (w602:T8)
      n207 = case shown="0" w600 {
        tunnel: w602 -> [w607 w623]
        tunnel: [w606 w622] -> w601
        frame 0 {
          w603 = FALSE  # Use Latest Calib
          n208 = Unbundle By Name(w607) -> ("Calib filename"=w609:path, "Ref Instrument type"=w605:T3)
          n209 = case shown="\"LDA\"" w605 {
            tunnel: [Inst_type."Propeller anemometer" ("Inst type") Inst_type."Pressure Transducer" ("Inst type") Inst_type."Pressure Transducer" ("Inst type") Inst_type."Pitot-static tube" ("Inst type") Inst_type."Preston tube" ("Inst type") Inst_type."Generic Linear" ("Inst type") Inst_type."Generic Polynomial" ("Inst type") Inst_type."Thermocouple" ("Inst type") Inst_type."Raw voltage" ("Inst type") Inst_type."Raw voltage" ("Inst type") Inst_type."Raw voltage" ("Inst type")] -> w604
            frame "Propellor anemometer" {
            }
            frame "Pressure Transducer" {
            }
            frame "Raw voltage" {
            }
            frame "Pitot-static tube" {
            }
            frame "Preston tube" {
            }
            frame "Generic Linear" {
            }
            frame "Generic Polynomial" {
            }
            frame "Thermocouple" {
            }
            frame "LDA" {
            }
            frame "Enter Value" {
            }
            frame "ADAM Channel" {
            }
          }
          n210 = call "Find_calibration_file.vi"("Inst type"=w604, "Use Latest Calib"=w603, "filename"=w609) -> ("filename out"=w608:path)  [unwired: 1 in]
          n211 = Bundle By Name(cluster=w607, "Calib filename"=w608) -> (w606:T8)
        }
        frame 1, Default {
          n212 = Bundle By Name(cluster=w623, "Calib filename"=path "") -> (w622:T8)
        }
      }
      n213 = local write "Ref vel for angle calib"(w601) -> ()
    }
    frame #7 {
      w630 = Ref_Inst_type."ADAM Channel" ("Ref Instrument type")
      n214 = local read "Ref vel for angle calib"() -> (w632:T8)
      n215 = global write "Calib_global.vi" "Ref Instrument type"(w627) -> ()
      n216 = property on="Ref vel for angle calib" class="Clust (strict)"() -> ("Disabled"=w625:u8)  [unwired: 2 in, 2 out]
      n217 = Unbundle By Name(w632) -> ("Ref Instrument type"=w631:T3)
      n218 = Equal To 0?(x=w625) -> (x = 0?=w624:bool)
      n219 = Equal?(x=w627, y=w630) -> (x = y?=w629:bool)
      n220 = local read "2nd ref instrument"() -> (w633:T7)
      n221 = Bundle By Name(cluster=w633, "2nd Ref type"=w631, "2nd inst present"=w624) -> (→"2nd ref instrument":T7)
      n222 = case shown="True" w624 {
        tunnel: w631 -> [_ w639]
        tunnel: w630 -> [_ w638]
        tunnel: w629 -> [w634 w636]
        tunnel: [w634 w635] -> w628
        frame False {
        }
        frame True {
          n223 = Equal?(x=w639, y=w638) -> (x = y?=w637:bool)
          n224 = Or(x=w637, y=w636) -> (x .or. y?=w635:bool)
        }
      }
    }
    frame #8 {
      n225 = Equal?(x=Calib_mode."Show Setup" ("Mode"), y=w647) -> (x = y?=w646:bool)
      n226 = And(x=w646, y=w645) -> (x .and. y?=w644:bool)
      n227 = global read "Calib_global.vi" "Pre Setup String"() -> (w643:string)
      n228 = case shown="True" w644 {
        tunnel: [w650 w656] -> w648
        tunnel: w643 -> [w652 w655]
        tunnel: "ADAM Channel name" -> [w651 w654]
        tunnel: [w649 w653] -> w641
        frame False {
          n229 = call "Get_Characters_from_string.vi"("Input string"=w652, "Variable name"=w651) -> ("Value"=w649:string)  [unwired: 1 in, 1 out]
          n230 = call "Characters_to_string.vi"("Characters to write"=w649, "Label for characters"=w651) -> ("Output string"=w650:string)
        }
        frame True {
          n231 = stacked-sequence {
            seq-local: [_ w660 _ _ _ _] -> [_ _ _ w670 _ _]
            seq-local: [_ _ _ w664 _ _] -> [_ _ _ _ _ _]
            seq-local: [_ _ w662 _ _ _] -> [_ _ _ _ _ w680]
            tunnel: [_ _ _ _ _ w679] -> w656
            tunnel: w655 -> [_ _ _ _ _ w675]
            tunnel: w654 -> [_ _ _ _ _ w674]
            tunnel: [_ _ _ _ _ w673] -> w653
            frame #0 {
              n232 = property on="Message" class="Str"("Visible"=TRUE) -> ()  [unwired: 2 in, 2 out]
              "Message" <- "Message\n\nCurrently trying to connect to the server.\n\nPlease Wait"
            }
            frame #1 {
              n233 = Get Date/Time In Seconds() -> (seconds since 1Jan1904=w659:timestamp)
              n234 = To Double Precision Float(number=w659) -> (double precision float=w660:dbl)
            }
            frame #2 {
              n235 = call "Get_ADAM_Ch_names_client.vi"("Channel names set"=Channel_names."Active Only") -> ("Ch names"=w662:string[])
            }
            frame #3 {
              n236 = Get Date/Time In Seconds() -> (seconds since 1Jan1904=w663:timestamp)
              n237 = To Double Precision Float(number=w663) -> (double precision float=w669:dbl)
              n238 = Subtract(x=w669, y=w670) -> (x-y=w668:dbl)
              n239 = Number To Decimal String(number=w668) -> (decimal integer string=w666:string)  [unwired: 1 out]
              n240 = Concatenate Strings("Server took ", w666, " Seconds to respond") -> (w664:string)
            }
            frame #4 {
              n241 = property on="Message" class="Str"("Visible"=FALSE) -> ()  [unwired: 2 in, 2 out]
            }
            frame #5 {
              n242 = call "Get_Characters_from_string.vi"("Input string"=w675, "Variable name"=w674) -> ("Status"=w678:enum16{"Char in string", "Char not in string"}, "Value"=w677:string)  [unwired: 1 in]
              n243 = case shown="\"Char in string\"" w678 {
                tunnel: w677 -> [w681 _]
                tunnel: [w681 "" ("Value")] -> w676
                frame "Char in string" {
                }
                frame "Char not in string" {
                }
              }
              n244 = call "Select_Single_ADAM_Ch.vi"("Desired Ch name (in)"=w676, "Available Ch names"=w680, "Message"="Please Choose Reference Instrument") -> ("Ch Name"=w673:string)  [unwired: 3 out]
              n245 = call "Characters_to_string.vi"("Characters to write"=w673, "Label for characters"=w674) -> ("Output string"=w679:string)
            }
          }
        }
      }
      n246 = global write "Calib_global.vi" "ADAM Channel Name"(w641) -> ()
    }
    frame #9 {
      n247 = local read "2nd ref instrument"() -> (w689:T7)
      n248 = Equal?(x=Calib_mode."Show Setup" ("Mode"), y=w696) -> (x = y?=w695:bool)
      n249 = Unbundle By Name(w689) -> ("2nd Ref type"=w687:T3, "2nd inst present"=w685:bool)
      n250 = global read "Calib_global.vi" "Pre Setup String"() -> (w693:string)
      n251 = Equal?(x=Ref_Inst_type."ADAM Channel" ("2nd Ref type"), y=w687) -> (x = y?=w686:bool)
      n252 = And(x=w686, y=w685) -> (x .and. y?=w684:bool)
      n253 = And(x=w695, y=w684) -> (x .and. y?=w694:bool)
      n254 = case shown="True" w694 {
        tunnel: [w698 w704] -> w683
        tunnel: w693 -> [w700 w703]
        tunnel: "ADAM Channel name for 2nd Ref Instr" -> [w699 w702]
        tunnel: [w697 w701] -> w691
        frame False {
          n255 = call "Get_Characters_from_string.vi"("Input string"=w700, "Variable name"=w699) -> ("Value"=w697:string)  [unwired: 1 in, 1 out]
          n256 = call "Characters_to_string.vi"("Characters to write"=w697, "Label for characters"=w699) -> ("Output string"=w698:string)
        }
        frame True {
          n257 = stacked-sequence {
            seq-local: [_ w708 _ _ _ _] -> [_ _ _ w718 _ _]
            seq-local: [_ _ _ w712 _ _] -> [_ _ _ _ _ _]
            seq-local: [_ _ w710 _ _ _] -> [_ _ _ _ _ w728]
            tunnel: [_ _ _ _ _ w727] -> w704
            tunnel: w703 -> [_ _ _ _ _ w723]
            tunnel: w702 -> [_ _ _ _ _ w722]
            tunnel: [_ _ _ _ _ w721] -> w701
            frame #0 {
              n258 = local write "Message"("Message\n\nCurrently trying to connect to the server.\n\nPlease Wait") -> ()
              n259 = property on="Message" class="Str"("Visible"=TRUE) -> ()  [unwired: 2 in, 2 out]
            }
            frame #1 {
              n260 = Get Date/Time In Seconds() -> (seconds since 1Jan1904=w707:timestamp)
              n261 = To Double Precision Float(number=w707) -> (double precision float=w708:dbl)
            }
            frame #2 {
              n262 = call "Get_ADAM_Ch_names_client.vi"("Channel names set"=Channel_names."Active Only") -> ("Ch names"=w710:string[])
            }
            frame #3 {
              n263 = Get Date/Time In Seconds() -> (seconds since 1Jan1904=w711:timestamp)
              n264 = To Double Precision Float(number=w711) -> (double precision float=w717:dbl)
              n265 = Subtract(x=w717, y=w718) -> (x-y=w716:dbl)
              n266 = Number To Decimal String(number=w716) -> (decimal integer string=w714:string)  [unwired: 1 out]
              n267 = Concatenate Strings("Server took ", w714, " Seconds to respond") -> (w712:string)
            }
            frame #4 {
              n268 = property on="Message" class="Str"("Visible"=FALSE) -> ()  [unwired: 2 in, 2 out]
            }
            frame #5 {
              n269 = call "Get_Characters_from_string.vi"("Input string"=w723, "Variable name"=w722) -> ("Status"=w726:enum16{"Char in string", "Char not in string"}, "Value"=w725:string)  [unwired: 1 in]
              n270 = case shown="\"Char in string\"" w726 {
                tunnel: w725 -> [w729 _]
                tunnel: [w729 "" ("Value")] -> w724
                frame "Char in string" {
                }
                frame "Char not in string" {
                }
              }
              n271 = call "Select_Single_ADAM_Ch.vi"("Desired Ch name (in)"=w724, "Available Ch names"=w728, "Message"="Please Choose 2nd Ref Channel") -> ("Ch Name"=w721:string)  [unwired: 3 out]
              n272 = call "Characters_to_string.vi"("Characters to write"=w721, "Label for characters"=w722) -> ("Output string"=w727:string)
            }
          }
        }
      }
      n273 = global write "Calib_global.vi" "ADAM Channel Name Vel Ref"(w691) -> ()
    }
    frame #10 {
      n274 = local read "Reference instrument"() -> (w735:T8)
      n275 = local read "2nd ref instrument"() -> (w736:T7)
      n276 = local read "Sampling speeds Output"() -> (w732:T6)
      n277 = local read "Abs Press (mbar)"() -> (w733:dbl)
      n278 = local read "Temp (deg C)"() -> (w731:dbl)
      n279 = global write "Calib_global.vi" "2nd ref instrument"(w736) -> ()
      n280 = Unbundle By Name(w732) -> ("Sampling Rate /ch (Hz)"=w738:sgl, "Samples /ch"=w739:i32)
      n281 = global write "Calib_global.vi" "Abs Press (mbar)"(w733) -> ()
      n282 = global write "Calib_global.vi" "Temp (deg C)"(w731) -> ()
      n283 = call "Calib_General_Setup.vi"("Reference instrument"=w735, "Requested No of samples"=w739, "Sampling rate (Hz)"=w738, "2nd ref instrument"=w736, "Temp"=w731, "Abs Press (mbar)"=w733) -> ("Output string"=w737:string, "LDA Data"=w734:bool)  [unwired: 8 out]
    }
    frame #11 {
      n284 = local read "Ref vel for angle calib"() -> (w748:T8)
      n285 = local read "Reference instrument"() -> (w747:T8)
      n286 = local read "Instrument type"() -> (w746:T9)
      n287 = global write "Calib_global.vi" "Instrument type"(w746) -> ()
      n288 = case shown="\"Propeller anemometer\", Default" w746 {
        tunnel: [w751 w752 w754] -> w745
        tunnel: w748 -> [w750 w753 _]
        tunnel: [w750 w753 w754] -> w741
        tunnel: w747 -> [w751 w752 w754]
        frame "Propeller anemometer", Default {
        }
        frame "Cross wire angle" {
        }
        frame "Cross wire velocity" {
        }
      }
      n289 = call "Reference_Inst_Info_2_string.vi"("Reference instrument"=w745, "Reference Name"="Reference instrument") -> ("Setup String"=w743:string)
      n290 = call "Reference_Inst_Info_2_string.vi"("Reference instrument"=w741, "Reference Name"="Ref vel for angle calib") -> ("Setup String"=w740:string)
      n291 = Concatenate Strings(w743, w740) -> (w749:string)
    }
    frame #12 {
      n292 = local read "Instrument type"() -> (w755:T9)
      n293 = case shown="\"Pulsed Wire\"" w755 {
        tunnel: ["" w764] -> w756
        tunnel: w757 -> [_ w763]
        frame "Propeller anemometer", Default {
        }
        frame "Pulsed Wire" {
          w759 = FALSE  # Check Calib file?
          n294 = case shown="\"Refit Curve\", Default" w763 {
            tunnel: [w766 w768] -> w762
            tunnel: [w765 w767] -> w761
            frame "Refit Curve", Default {
              w766 = FALSE  # Show Panel?
              w765 = T12 TRUE  # OK
            }
            frame "Show Setup" {
              w768 = TRUE  # Show Panel?
              w767 = T12 FALSE  # OK
            }
          }
          n295 = global read "Calib_global.vi" "Pre Setup String"() -> (w760:string)
          n296 = call "PWA_Setup_Panel.vi"("Show Panel?"=w762, "Check Calib file?"=w759, "OK"=w761, "Incoming Setup String"=w760) -> ("Outgoing Setup String"=w764:string)  [unwired: 3 out]
        }
      }
    }
    frame #13 {
      n297 = local read "instrument to calibrate"() -> (w771:T11)
      n298 = for {
        tunnel: w771 -> [w802] mode=indexing
        shift-right: [w787] -> w774
        shift-left: "" -> [w791]
        i -> [w801]
        n299 = Unbundle By Name(w802) -> ("high limit (10V)"=w798:sgl, "low limit (-10V)"=w793:sgl, "Ch No"=w792:i16, "DAQmx Channel"=w780:tag)
        n300 = Increment(x=w801) -> (x+1=w786:i32)
        n301 = Format Into String(format string="Inst_to_calibrate_element_%d ", w786) -> (resulting string=w781:string)  [unwired: 2 in, 1 out]
        n302 = Concatenate Strings(w781, "Low limit") -> (w797:string)
        n303 = Concatenate Strings(w781, "Ch No") -> (w796:string)
        n304 = Concatenate Strings(w781, "DAQ Ch") -> (w782:string)
        n305 = Concatenate Strings(w781, "High limit") -> (w799:string)
        n306 = call "Characters_to_string.vi"("Characters to write"=w780, "Label for characters"=w782) -> ("Output string"=w784:string)
        n307 = call "Value_to_string.vi"("Value"=w793, "Label for value"=w797) -> ("Output string"=w789:string)  [unwired: 1 in]
        n308 = call "Value_to_string.vi"("Value"=w792, "Label for value"=w796) -> ("Output string"=w788:string)  [unwired: 1 in]
        n309 = call "Value_to_string.vi"("Value"=w798, "Label for value"=w799) -> ("Output string"=w790:string)  [unwired: 1 in]
        n310 = Concatenate Strings(w791, w790, w789, w788, w784) -> (w787:string)
      }
      n311 = Array Size(array=w771) -> (size(s)=w770:i32)
      n312 = Equal To 0?(x=w770) -> (x = 0?=w769:bool)
      n313 = case shown="True" w769 {
        tunnel: [w776 i16 -10 ("Ch No")] -> w772
        tunnel: w771 -> [w775 _]
        frame False {
          w778 = 0  # index
          n314 = Index Array(array=w775, index=w778) -> (element=w777:T18)
          n315 = Unbundle By Name(w777) -> ("Ch No"=w776:i16)
        }
        frame True {
        }
      }
      n316 = global write "Calib_global.vi" "Calib Ch No"(w772) -> ()
    }
    frame #14 {
      n317 = local read "Preston tube diammeter in mm"() -> (w806:dbl)
      n318 = local read "Instrument type"() -> (w817:T9)
      n319 = property on="Instrument type" class="Enum (strict)"() -> ("Strings []"=w818:string[])  [unwired: 2 in, 2 out]
      n320 = local read "angle calib"() -> (w811:T10)
      n321 = property on="angle calib" class="Enum (strict)"() -> ("Strings []"=w812:string[])  [unwired: 2 in, 2 out]
      n322 = Index Array(array=w818, index=w817) -> (element=w816:string)
      n323 = Index Array(array=w812, index=w811) -> (element=w810:string)
      n324 = call "Characters_to_string.vi"("Characters to write"=w816, "Label for characters"="Instrument_type_to Calibrate") -> ("Output string"=w814:string)
      n325 = call "Value_to_string.vi"("Value"=w806, "Label for value"="Preston tube diameter in mm" ("Variable name")) -> ("Output string"=w805:string)  [unwired: 1 in]
      n326 = call "Characters_to_string.vi"("Characters to write"=w810, "Label for characters"="Angle calib") -> ("Output string"=w809:string)
      n327 = local read "Fixed n out"() -> (w822:bool)
      n328 = Concatenate Strings(w805, w814, w809) -> (w829:string)
      n329 = Select(t="TRUE", s=w822, f="FALSE") -> (s? t:f=w823:string)
      n330 = global read "Calib_global.vi" "New Setup String"() -> (w821:string)
      n331 = call "Characters_to_string.vi"("Characters to write"=w823, "Label for characters"="Fixed Coefficient n") -> ("Output string"=w819:string)
      n332 = Concatenate Strings(w821, w819, w829, w828, w803, w827, w804, w820, w808) -> (w830:string)
      n333 = global write "Calib_global.vi" "New Setup String"(w830) -> ()
    }
    frame #15 {
      n334 = Equal?(x=Calib_mode."Show Setup" ("Mode"), y=w836) -> (x = y?=w835:bool)
      n335 = And(x=w834, y=w835) -> (x .and. y?=w833:bool)
      n336 = case shown="True" w833 {
        tunnel: [FALSE ("Synchronise with LDA") FALSE ("Synchronise with LDA")] -> w831
        frame False {
        }
        frame True {
          n337 = global read "LDA_meas_global_1.vi" "BSA Type"() -> (w840:T19)
          n338 = case shown="\"BSA F60\"" w840 {
            tunnel: TRUE -> [_ w850]
            frame "57N11" {
              n339 = stacked-sequence {
                frame #0 {
                  n340 = Bundle By Name(cluster=T16 {"dimensions"=enum."2D", "Analogue Freq Multiplier"=0.1} ("LDA set up"), "dimensions"=enum16{"1D", "2D"}."1D", "Analogue Freq Multiplier"=2.0) -> (w843:T16)
                  n341 = global write "Meas_global.vi" "LDA set up"(w843) -> ()
                }
                frame #1 {
                  w845 = "1"  # BSA Number
                  n342 = call "Control_BSA_setup.vi"("setup"=Setup."Show Setup", "BSA number"=w845) -> ()  [unwired: 14 out]
                }
                frame #2 {
                  n343 = global read "LDA_meas_global_2.vi" "BSA2 info"() -> (w847:T20)
                  n344 = Unbundle By Name(w847) -> ("GPIB Address"=w848:string)
                  n345 = call "Set_BSA_Coincidence.vi"("GPIB address"=w848, "Set Coincidence"=enum16{"Slave", "Master", "Private"}."Slave") -> ()  [unwired: 1 in, 5 out]
                }
              }
            }
            frame "BSA F60" {
              n346 = disable-structure shown="TARGET_TYPE==Windows" {
                disable-tunnel: w850 -> [_ w851]
                frame condition #0 {
                }
                frame condition #1 (active) {
                  n347 = call "Edit_BSA_IP.vi"("Show Panel"=w851) -> ()  [unwired: 3 out]
                }
              }
            }
          }
        }
      }
      n348 = global write "Meas_global.vi" "Synchronise with LDA"(w831) -> ()
    }
    frame #16 {
      w860 = TRUE  # Lock File
      w869 = FALSE  # advisory dialog? (display:T)
      w870 = FALSE  # append to file? (new file:F)
      n349 = local read "Ch & Spans"() -> (w852:T1[])
      n350 = local read "Calib filename"() -> (w871:path)
      n351 = local read "Instrument type"() -> (w858:T9)
      n352 = global read "Meas_global.vi" "LDA data"() -> (w863:enum16{"No LDA data", "Take LDA data"})
      n353 = global write "Calib_global.vi" "Ref Calib file"(w871) -> ()
      n354 = case shown="\"Take LDA data\"" w863 {
        tunnel: ["" w880] -> w861
        frame "No LDA data" {
        }
        frame "Take LDA data" {
          w879 = ""  # Used to be LDA-header.vi
          n355 = call "LDA_U16_data_header.vi"() -> ("Output string"=w881:string)  [unwired: 1 out]
          n356 = Concatenate Strings(w879, w881) -> (w880:string)
        }
      }
      n357 = case shown="\"Pulsed Wire\"" w858 {
        tunnel: ["" w873] -> w857
        frame "Propeller anemometer", Default {
        }
        frame "Pulsed Wire" {
          n358 = property on="PWA Data" class="Enum (strict)"() -> ("Strings []"=w876:string[])  [unwired: 2 in, 2 out]
          n359 = Index Array(array=w876, index=PWA_Data."One Ch PWA" ("PWA Data")) -> (element=w874:string)
          n360 = call "Characters_to_string.vi"("Characters to write"=w874, "Label for characters"="Pulsed_Wire_Data" ("Variable name")) -> ("Output string"=w873:string)
        }
      }
      n361 = call "Calib_Ch_setup.vi"("Preston tube diammeter in mm"="Preston tube diammeter in mm", "Ch & Spans"=w852, "Calib filename"=w871) -> ("Output string"=w864:string)
      n362 = global write "Calib_global.vi" "Ch & Spans"(w852) -> ()
      n363 = call "Date_and_Time_to_string.vi"() -> ("Date and time (spreadsheet)"=w862:string)
      n364 = Concatenate Strings(w862, w857, w861, w865, w864, w856) -> (w866:string)
      n365 = call "Setup_Filepath.vi"("Setup File Type"=Setup_Filetype."Measurement Setups", "Filename in"="Calib_Setup.xls") -> ("Filename Out"=w853:path)  [unwired: 1 out]
      n366 = call "Add_label_to_string.vi"("String to write"=w866, "File Label"="Raw data header") -> ("Output string"=w867:string)
      n367 = call "Write_Characters_To_File.vi"("file path (dialog if empty)"=w853, "advisory dialog? (display:T)"=w869, "character string"=w867, "append to file? (new file:F)"=w870, "Lock File"=w860) -> ()  [unwired: 4 out]
    }
    frame #17 {
      n368 = case shown="\"Show Setup\"" w882 {
        frame "Show Setup" {
          n369 = Current VI's Path() -> (path=w884:path)
          n370 = call "Open_Close_Front_Panel.ph.vi"("Front Panel Window:Open"=FALSE, "VI path"=w884) -> ()  [unwired: 2 out]
        }
        frame "Take a New Calibration Point", Default {
        }
      }
    }
  }
